vi "ControlsToCluster.vi"(10 "Path (px)":cluster{dbl, dbl}[](array[cluster]), 11 "Path (in)":cluster{dbl, dbl}[](array[cluster])) -> (3 "Path File Data":T1={"RobotNeeded"={"Path"=[], "MaxVel"=0.0, "MaxAccel"=0.0, "Backwards?"=FALSE, "PointSpacing"=0.0, "LookaheadDist"=0.0, "Speed/Curve"=1.8, "SlowDistanceAtEnd"=12.0, "SlowSpeed"=15.0, "MaxDeAccel"=0.0}, "Meta"={"Path (px)"=[], "RobotWidth"=0.0, "RobotLength"=0.0, "CenterOfRotYOffset"=0.0, "Roundedness"=0.0, "StartingPositionPreset"=0}} {"RobotNeeded"."SlowSpeed" format="%#_13g"; "RobotNeeded"."SlowDistanceAtEnd" format="%#_13g"; "RobotNeeded"."Speed/Curve" format="%#_13g"})   [LabVIEW 2019]
uses:
  Dawgma Programming Library/Controls/PurePursuit/PathFileData.ctl
  Dawgma Programming Library/Controls/PurePursuit/RobotNeededPathData.ctl
  Robot Project/Configuration/Constants.vi
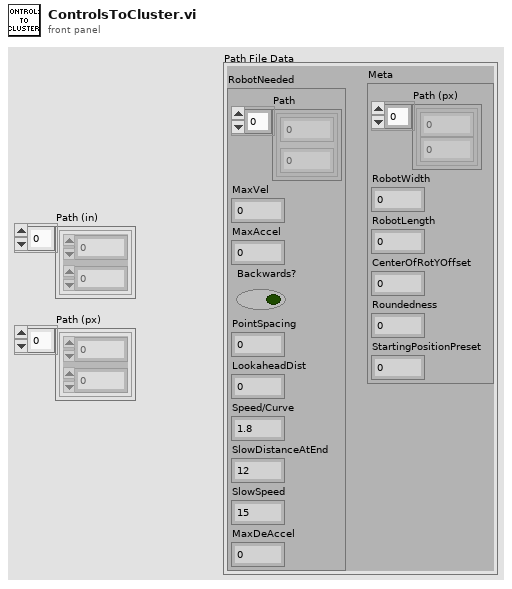
[diagram p1: front panel]
types:
  T1 = typedef "PathFileData.ctl" = cluster{"RobotNeeded":T2, "Meta":cluster{"Path (px)":cluster{i32, i32}[], "RobotWidth":dbl, "RobotLength":dbl, "CenterOfRotYOffset":dbl, "Roundedness":dbl, "StartingPositionPreset":u32}}
  T2 = typedef "RobotNeededPathData.ctl" = cluster{"Path":cluster{dbl, dbl}[], "MaxVel":dbl, "MaxAccel":dbl, "Backwards?":bool, "PointSpacing":dbl, "LookaheadDist":dbl, "Speed/Curve":dbl, "SlowDistanceAtEnd":dbl, "SlowSpeed":dbl, "MaxDeAccel":dbl}
  T3 = cluster{"Path (px)":cluster{i32, i32}[], "RobotWidth":dbl, "RobotLength":dbl, "CenterOfRotYOffset":dbl, "Roundedness":dbl, "StartingPositionPreset":u32, "PathName":string}
  T4 = cluster{"Path (px)":cluster{i32, i32}[], "RobotWidth":dbl, "RobotLength":dbl, "CenterOfRotYOffset":dbl, "Roundedness":dbl, "StartingPositionPreset":u32}
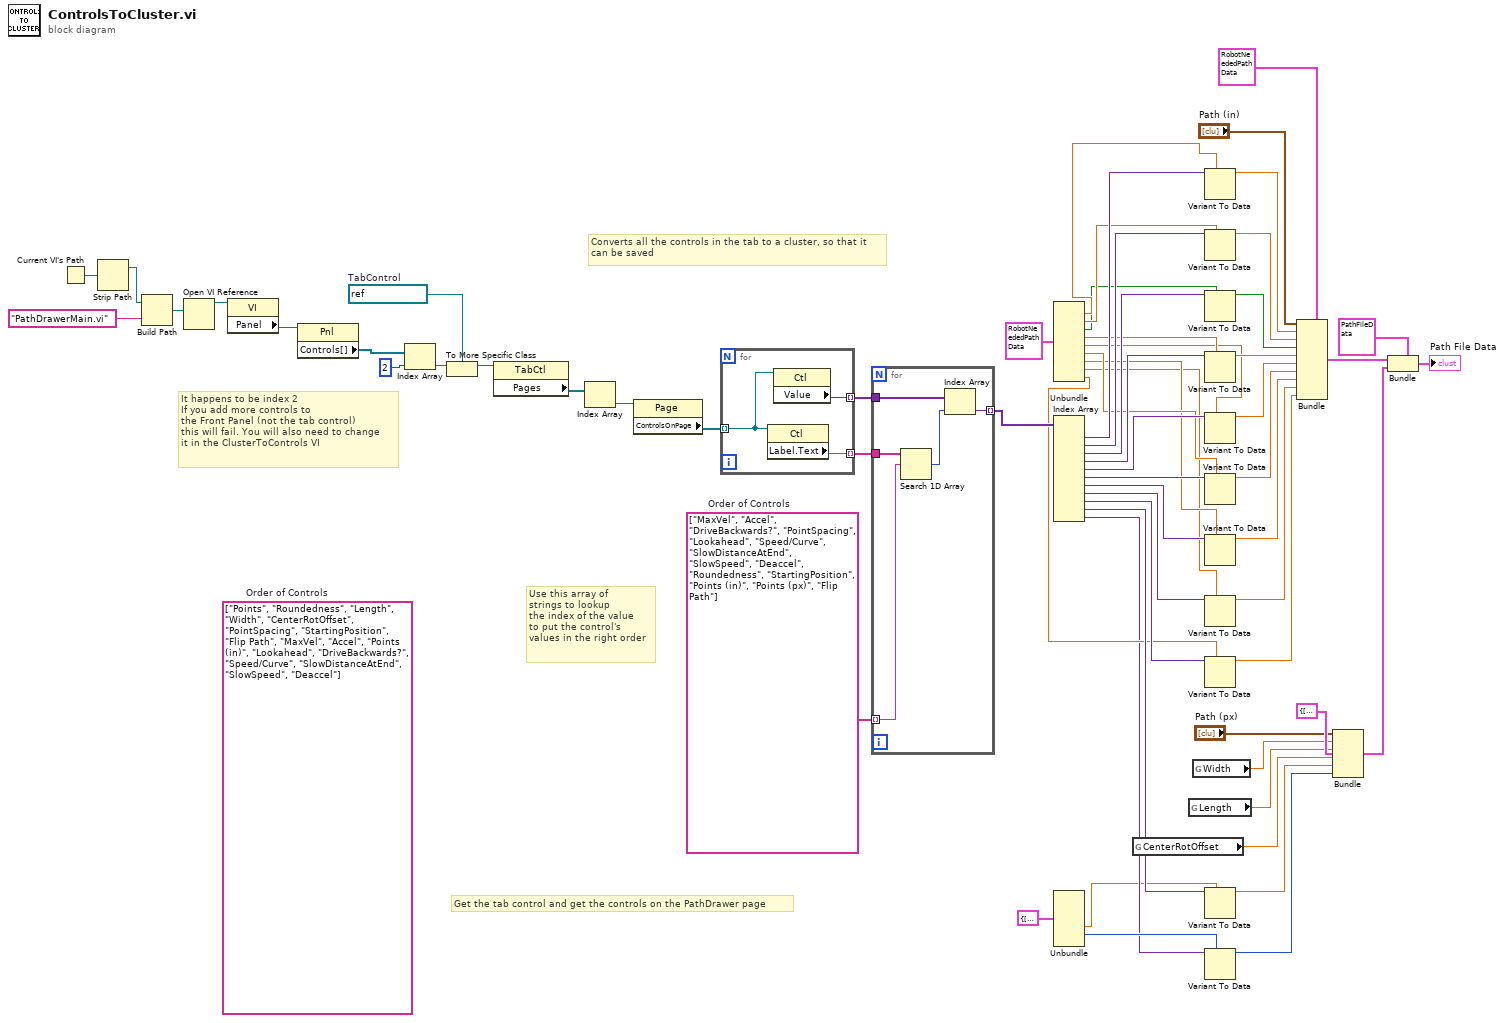
[diagram p0: block diagram]
diagram:
  w41 = string[] ["MaxVel", "Accel", "DriveBackwards?", "PointSpacing", "Lookahead", "Speed/Curve", "SlowDistanceAtEnd", "SlowSpeed", "Deaccel", "Roundedness", "StartingPosition", "Points (in)", "Points (px)", "Flip Path"]  # Order of Controls
  (unwired) string[] ["Points", "Roundedness", "Length", "Width", "CenterRotOffset", "PointSpacing", "StartingPosition", "Flip Path", "MaxVel", "Accel", "Points (in)", "Lookahead", "DriveBackwards?", "Speed/Curve", "SlowDistanceAtEnd", "SlowSpeed", "Deaccel"]  # Order of Controls
  w63 = refnum<vi> refnum  # TabControl
  # "Converts all the controls in the tab to a cluster, so that it\ncan be saved"
  # "Use this array of\nstrings to lookup\nthe index of the value\nto put the control's\nvalues in the right order"
  # "It happens to be index 2\nIf you add more controls to\nthe Front Panel (not the tab control)\nthis will fail. You will also need to change\nit in the ClusterToControls VI"
  # "Get the tab control and get the controls on the PathDrawer page"
  n1 = Current VI's Path() -> (path=w12:path)
  n2 = Strip Path(path=w12) -> (stripped path=w11:path)  [unwired: 1 out]
  n3 = Build Path(base path=w11, name or relative path="PathDrawerMain.vi") -> (appended path=w9:path)
  n4 = Open VI Reference(vi path=w9) -> (vi reference=w8:refnum<vi>)  [unwired: 5 in, 1 out]
  n5 = property class="VI"(reference=w8) -> ("Panel"=w13:refnum<vi>)  [unwired: 1 in, 2 out]
  n6 = property class="Pnl"(reference=w13) -> ("Controls[]"=w7:refnum<vi>[])  [unwired: 1 in, 2 out]
  n7 = Index Array(array=w7, index=2) -> (element=w62:refnum<vi>)
  n8 = To More Specific Class(target class=w63, reference=w62) -> (specific class reference=w61:refnum<vi>)  [unwired: 1 in, 1 out]
  n9 = property class="TabCtl"(reference=w61) -> ("Pages"=w60:refnum<vi>[])  [unwired: 1 in, 2 out]
  n10 = Index Array(array=w60) -> (element=w59:refnum<vi>)  [unwired: 1 in]
  n11 = property class="Page"(reference=w59) -> ("ControlsOnPage"=w58:refnum<vi>[])  [unwired: 1 in, 2 out]
  n12 = for {
    tunnel: w58 -> [w66] mode=indexing
    tunnel: [w67] -> w42 mode=indexing
    tunnel: [w65] -> w43 mode=indexing
    n13 = property class="Ctl"(reference=w66) -> ("Label.Text"=w67:string)  [unwired: 1 in, 2 out]
    n14 = property class="Ctl"(reference=w66) -> ("Value"=w65:variant)  [unwired: 1 in, 2 out]
  }
  n15 = for {
    tunnel: [w68] -> w44 mode=indexing
    tunnel: w43 -> [w70]
    tunnel: w42 -> [w72]
    tunnel: w41 -> [w71] mode=indexing
    n16 = Search 1D Array(1D array=w72, element=w71) -> (index of element=w69:i32)  [unwired: 1 in]
    n17 = Index Array(array=w70, index=w69) -> (element=w68:variant)
  }
  n18 = Unbundle(T2 {"Path"=[], "MaxVel"=0.0, "MaxAccel"=0.0, "Backwards?"=FALSE, "PointSpacing"=0.0, "LookaheadDist"=0.0, "Speed/Curve"=1.8, "SlowDistanceAtEnd"=12.0, "SlowSpeed"=15.0, "MaxDeAccel"=0.0} ("RobotNeededPathData")) -> ("MaxVel"=w40:dbl, "MaxAccel"=w38:dbl, "Backwards?"=w35:bool, "PointSpacing"=w34:dbl, "LookaheadDist"=w31:dbl, "Speed/Curve"=w30:dbl, "SlowDistanceAtEnd"=w28:dbl, "SlowSpeed"=w25:dbl, "MaxDeAccel"=w24:dbl)  [unwired: 1 out]
  n19 = Index Array(array=w44) -> (element #1=w57:variant, element #2=w56:variant, element #3=w55:variant, element #4=w54:variant, element #5=w53:variant, element #6=w52:variant, element #7=w51:variant, element #8=w50:variant, element #9=w49:variant, element #10=w48:variant, element #11=w6:variant)  [unwired: 11 in]
  n20 = Unbundle(T3 {"Path (px)"=[], "RobotWidth"=0.0, "RobotLength"=0.0, "CenterOfRotYOffset"=0.0, "Roundedness"=0.0, "StartingPositionPreset"=0, "PathName"=""} ("Meta")) -> ("Roundedness"=w3:dbl, "StartingPositionPreset"=w17:u32)  [unwired: 5 out]
  n21 = global read "Constants.vi" "CenterRotOffset"() -> (w4:dbl)
  n22 = global read "Constants.vi" "Length"() -> (w5:dbl)
  n23 = global read "Constants.vi" "Width"() -> (w1:dbl)
  n24 = Variant To Data(type=w40, Variant=w57) -> (data=w39:dbl)  [unwired: 1 in, 1 out]
  n25 = Variant To Data(type=w38, Variant=w56) -> (data=w37:dbl)  [unwired: 1 in, 1 out]
  n26 = Variant To Data(type=w35, Variant=w55) -> (data=w36:bool)  [unwired: 1 in, 1 out]
  n27 = Variant To Data(type=w34, Variant=w54) -> (data=w33:dbl)  [unwired: 1 in, 1 out]
  n28 = Variant To Data(type=w31, Variant=w53) -> (data=w32:dbl)  [unwired: 1 in, 1 out]
  n29 = Variant To Data(type=w30, Variant=w52) -> (data=w29:dbl)  [unwired: 1 in, 1 out]
  n30 = Variant To Data(type=w28, Variant=w51) -> (data=w27:dbl)  [unwired: 1 in, 1 out]
  n31 = Variant To Data(type=w25, Variant=w50) -> (data=w26:dbl)  [unwired: 1 in, 1 out]
  n32 = Variant To Data(type=w24, Variant=w49) -> (data=w23:dbl)  [unwired: 1 in, 1 out]
  n33 = Variant To Data(type=w3, Variant=w48) -> (data=w2:dbl)  [unwired: 1 in, 1 out]
  n34 = Variant To Data(type=w17, Variant=w6) -> (data=w16:u32)  [unwired: 1 in, 1 out]
  n35 = Bundle(cluster=T2 {"Path"=[], "MaxVel"=0.0, "MaxAccel"=0.0, "Backwards?"=FALSE, "PointSpacing"=0.0, "LookaheadDist"=0.0, "Speed/Curve"=1.8, "SlowDistanceAtEnd"=12.0, "SlowSpeed"=15.0, "MaxDeAccel"=0.0} ("RobotNeededPathData"), "Path"="Path (in)", "MaxVel"=w39, "MaxAccel"=w37, "Backwards?"=w36, "PointSpacing"=w33, "LookaheadDist"=w32, "Speed/Curve"=w29, "SlowDistanceAtEnd"=w27, "SlowSpeed"=w26, "MaxDeAccel"=w23) -> (w15:T2)
  n36 = Bundle(cluster=T4 {"Path (px)"=[], "RobotWidth"=0.0, "RobotLength"=0.0, "CenterOfRotYOffset"=0.0, "Roundedness"=0.0, "StartingPositionPreset"=0} ("Meta"), "Path (px)"="Path (px)", "RobotWidth"=w1, "RobotLength"=w5, "CenterOfRotYOffset"=w4, "Roundedness"=w2, "StartingPositionPreset"=w16) -> (w21:T4)
  n37 = Bundle(cluster=T1 {"RobotNeeded"={"Path"=[], "MaxVel"=0.0, "MaxAccel"=0.0, "Backwards?"=FALSE, "PointSpacing"=0.0, "LookaheadDist"=0.0, "Speed/Curve"=1.8, "SlowDistanceAtEnd"=12.0, "SlowSpeed"=15.0, "MaxDeAccel"=0.0}, "Meta"={"Path (px)"=[], "RobotWidth"=0.0, "RobotLength"=0.0, "CenterOfRotYOffset"=0.0, "Roundedness"=0.0, "StartingPositionPreset"=0}} ("Data"), "RobotNeeded"=w15, "Meta"=w21) -> (→"Path File Data":T1)
